vi "Write Stepper Motor.vi"(10 "Stepper Motor":T1={"Maximum Step Rate"=2000.0} {"Maximum Step Rate" min=1.0 max=4000.0 format="%.3f"}, 11 "StepperMotor in":refnum<class "StepperMotor.lvclass">) -> (3 "StepperMotor out":refnum<class "StepperMotor.lvclass">)   [LabVIEW 2013, in "StepperMotor.lvlib" / "StepperMotor.lvclass"]
uses:
  <userlib>/Common/Devices/StepperMotor/StepperMotor/StepperMotor.lvclass
  <userlib>/Common/Devices/StepperMotor/Config/StepperMotor.ctl
  <userlib>/Common/Devices/StepperMotor/StepperMotor/StepperMotor.lvclass/StepperMotor.ctl
  <userlib>/Common/Devices/StepperMotor/StepperMotor.lvlib
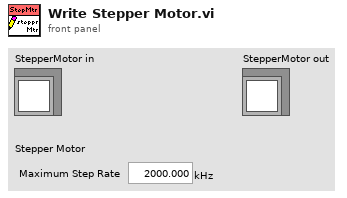
[diagram p1: front panel]
types:
  T1 = typedef "StepperMotor.lvlib/StepperMotor.ctl" = cluster{"Maximum Step Rate":dbl[unit]}
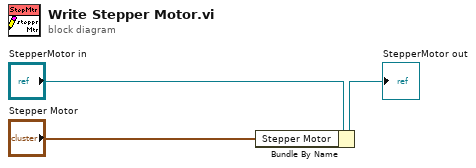
[diagram p0: block diagram]
diagram:
  n1 = Bundle By Name(cluster="StepperMotor in", "Stepper Motor"="Stepper Motor") -> (→"StepperMotor out":refnum<class "StepperMotor.lvclass">)
